vi "Main (Blink).vi"() -> ()   [LabVIEW 2018]
uses:
  <vilib>/Platform/TimedLoop/XDataNode/timing_clust.ctl
  <vilib>/Platform/TimedLoop/XDataNode/nitl_modes.ctl
  <vilib>/Platform/TimedLoop/XDataNode/wakeup.ctl
  <extravilib>/ChannelInstances/Tag-bool/Read With Abort.vi
  <extravilib>/ChannelInstances/Tag-bool/Write With Abort.vi
  <extravilib>/ChannelInstances/Tag-bool/Instantiate.vi
  <extravilib>/ChannelInstances/Tag-bool/EndpointRead.vi
  <extravilib>/ChannelInstances/Tag-bool/Endpoint.vi
  <vilib>/platform/TimedLoop/XDataNode/XDataNode.xnode
  <vilib>/Platform/TimedLoop/XDataNode/XDNodeRunTimeDep.lvlib
  <extravilib>/ChannelInstances/Tag-bool.lvlib
panel:
  out "SubVI 2":bool
  out "SubVI 1":bool
  out "Loop 2":bool
  out "Loop 1":bool
  in  "OK Button":bool
  # "Test Parallel Tasks"
  # "Blink LEDS at different frequencies.\nLEDs are written in parallel loops.\n\nSignal \"Stop\" by \"Tag channel\".\n\nLEDs are switched by SubVI as well.\n(reentrant and indicator passed by\nreference)."
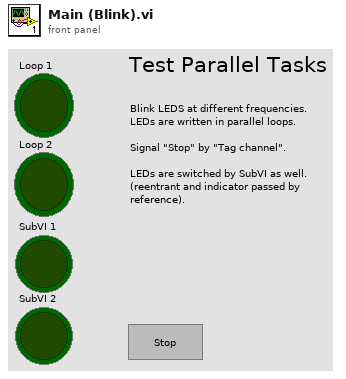
[diagram p1: front panel]
types:
  T1 = typedef "XDNodeRunTimeDep.lvlib/timing_clust.ctl" = cluster{"Expected End [f-1]":u64, "Actual End [f-1]":u64, "Finished Late? [f-1]":bool, "Expected End [i-1]":u64, "Actual End [i-1]":u64, "Finished Late? [i-1]":bool, "Expected Start [i]":u64, "Actual Start [i]":u64, "Expected Start [f]":u64, "Actual Start [f]":u64, "Source Name":string, "Structure Name":string, "Period":i64, "Deadline":i64, "Offset":i64, "Start":i64, "Priority":i32, "Timeout":i32, "Mode":T2, "Wakeup Reason":T3, "Error":errorcluster, "Source Type":string, "Secondary Source Type":string, "Global End Time":u64, "Global Start Time":u64, "Frame Duration":u64, "Iteration Duration":u64, "Assigned CPU":i32, "I/O Scan Engine Mode":u32}
  T2 = typedef "XDNodeRunTimeDep.lvlib/nitl_modes.ctl" = enum32{"No Change", "Process missed periods, maintain original phase", "Discard missed periods, maintain original phase", "Process missed periods, ignore original phase", "Discard missed periods, ignore original phase"}
  T3 = typedef "XDNodeRunTimeDep.lvlib/wakeup.ctl" = enum32{"Normal", "Aborted", "Asynchronous wakeup", "Timing source error", "Timed loop error", "Timeout"}
  T4 = typedef "Tag-bool.lvlib/))Channel.ctl" = refnum<queue>
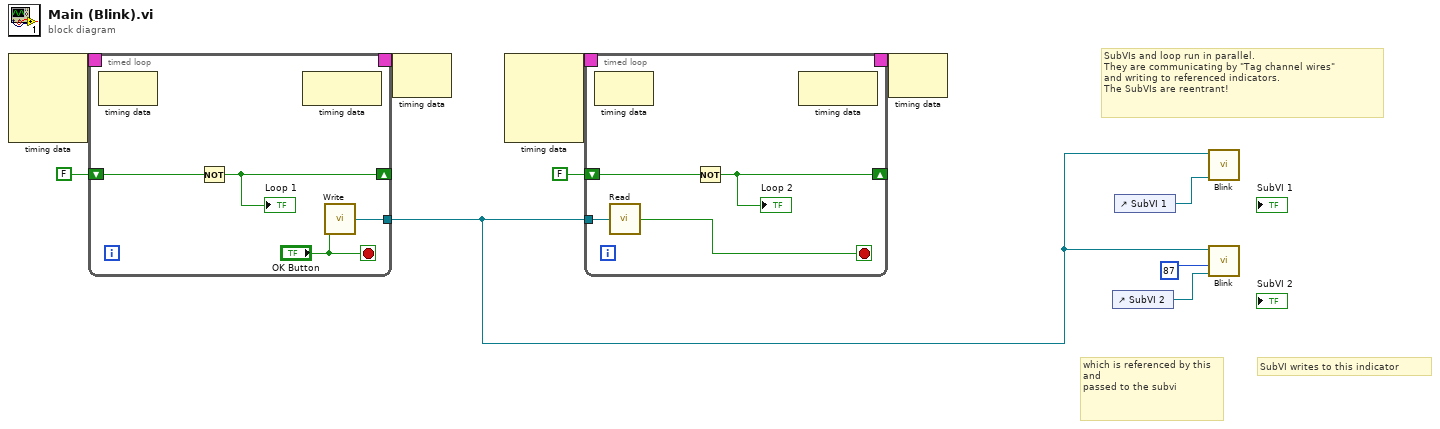
[diagram p0: block diagram]
diagram:
  # "SubVIs and loop run in parallel.\nThey are communicating by \"Tag channel wires\"\nand writing to referenced indicators.\nThe SubVIs are reentrant!"
  # "which is referenced by this and\npassed to the subvi"
  # "SubVI writes to this indicator"
  n1 = node-c288() -> (w10:T1)  [unwired: 4 in]
  n2 = timed-loop {
    timing: w10 -> [_]
    timing-out: [_] -> w9
    shift-right: [w13] -> _
    shift-left: FALSE -> [w14]
    tunnel: [w11] -> w4
    stop <- "OK Button" stop-if-true
    n3 = node-c288() -> ()  [unwired: 1 in, 1 out]
    n4 = Not(x=w14) -> (.not. x?=w13:bool)
    "Loop 1" <- w13
    n5 = node-c288() -> ()  [unwired: 1 in, 1 out]
    n6 = call <extravilib>:"Write.vi"("element"="OK Button") -> ("channel"=w11:T4)  [unwired: 1 out]
  }
  n7 = node-c288(w9) -> ()  [unwired: 1 out]
  n8 = node-c288() -> (w7:T1)  [unwired: 4 in]
  n9 = timed-loop {
    timing: w7 -> [_]
    timing-out: [_] -> w6
    shift-right: [w19] -> _
    shift-left: FALSE -> [w20]
    tunnel: w4 -> [w18]
    stop <- w17 stop-if-true
    n10 = node-c288() -> ()  [unwired: 1 in, 1 out]
    n11 = call <extravilib>:"Read.vi"("channel"=w18) -> ("element"=w17:bool)  [unwired: 1 in, 1 out]
    n12 = Not(x=w20) -> (.not. x?=w19:bool)
    "Loop 2" <- w19
    n13 = node-c288() -> ()  [unwired: 1 in, 1 out]
  }
  n14 = node-c288(w6) -> ()  [unwired: 1 out]
  n15 = control-ref of="SubVI 2"() -> (w3:refnum<vi>)
  n16 = control-ref of="SubVI 1"() -> (w2:refnum<vi>)
  n17 = call "Blink.vi"("Ctl Refnum"=w2, "Channel in"=w4) -> ()  [unwired: 10 in]
  n18 = call "Blink.vi"("Ctl Refnum"=w3, "Period"=i64 87, "Channel in"=w4) -> ()  [unwired: 9 in]
